vi "getAcquisitionSettings.vi"(8 "error in (no error)":errorcluster, 11 "CameraAcquisitor in":refnum<class "CameraAcquisitor.lvclass">) -> (0 "error out":errorcluster, 3 "CameraAcquisitor out":refnum<class "CameraAcquisitor.lvclass">)   [LabVIEW 2009, in "Hardware.lvlib" / "Channels.lvlib" / "CameraAcquisitor.lvclass"]
uses:
  CameraAcquisitor.lvclass
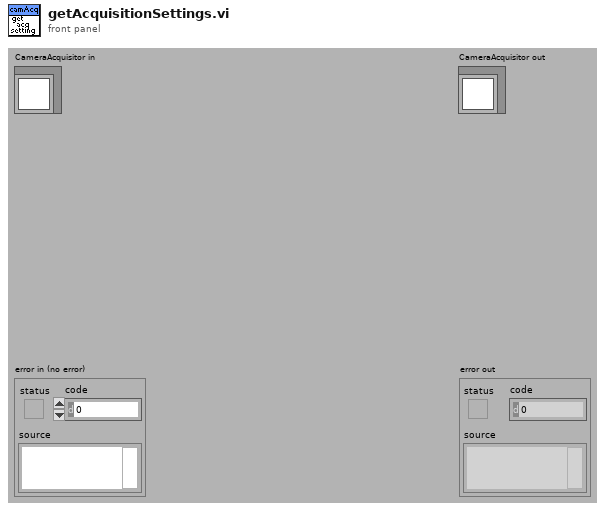
[diagram p1: front panel]
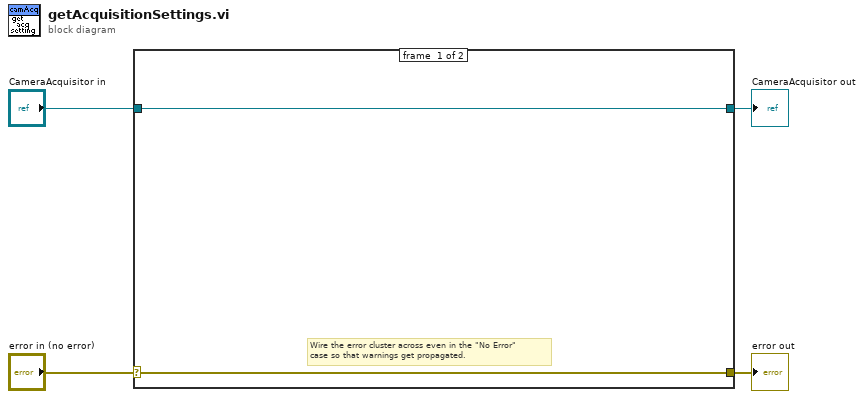
[diagram p0: block diagram]
diagram:
  n1 = case shown="No Error" "error in (no error)" {
    selector: "error in (no error)" -> [w5 w8]
    tunnel: [w5 w8] -> w3
    tunnel: [w6 w7] -> w1
    tunnel: "CameraAcquisitor in" -> [w6 w7]
    frame #0 {
      # "Wire the error cluster across even in the \"No Error\"\ncase so that warnings get propagated."
    }
    frame #1 {
    }
  }
  "error out" <- w3
  "CameraAcquisitor out" <- w1
